vi "33120PRF.vi"(0 "VISA session in":refnum<visa-resource-name>, 2 "Prf (kHz)":dbl format="%.2f", 3 "error in (no error)":errorcluster) -> (5 "VISA session out":refnum<visa-resource-name>, 6 "PRF (kHz)":dbl format="%.2f", 8 "error out":errorcluster)   [LabVIEW 2022 SP3]
uses:
  Pulsers/PulserGlobals.vi
panel:
  # "Set up to work with HP33120A. To set the PRF"
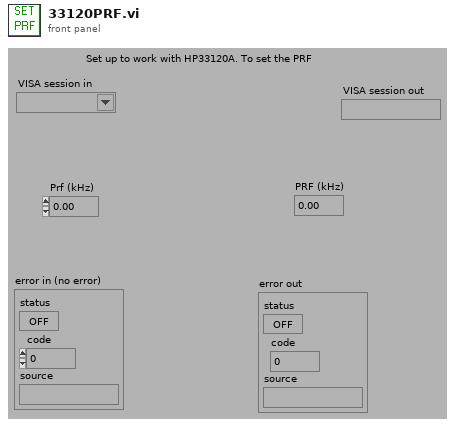
[diagram p1: front panel]
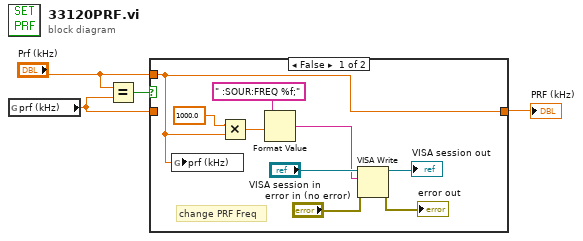
[diagram p0: block diagram]
diagram:
  n1 = global read "PulserGlobals.vi" "prf (kHz)"() -> (w1:dbl)
  n2 = Equal?(x="Prf (kHz)", y=w1) -> (x = y?=w4:bool)
  n3 = case shown="False" w4 {
    tunnel: [w5 w14] -> w2
    tunnel: w1 -> [_ w14]
    tunnel: "Prf (kHz)" -> [w5 _]
    frame False {
      # "change PRF Freq"
      n4 = global write "PulserGlobals.vi" "prf (kHz)"(w5) -> ()
      n5 = Multiply(x=1000.0, y=w5) -> (x*y=w12:dbl)
      n6 = Format Value(format string=" :SOUR:FREQ %f;", value (0)=w12) -> (output string=w6:string)  [unwired: 1 out]
      n7 = VISA Write(VISA resource name="VISA session in", write buffer=w6, error in (no error)="error in (no error)") -> (VISA resource name out=→"VISA session out":refnum<visa-resource-name>, error out=→"error out":errorcluster)  [unwired: 1 out]
    }
    frame True {
    }
  }
  "PRF (kHz)" <- w2
